vi "SetGXMLCfgRTD.vi"(8 "error in (no error)":errorcluster, 10 "RTDChanCfg":T1, 11 "RTD in":refnum<class "RTD.lvclass">) -> (0 "error out":errorcluster, 3 "RTD out":refnum<class "RTD.lvclass">)   [LabVIEW 2012, in "Measurement Channels.lvlib" / "RTD.lvclass"]
uses:
  RTD.lvclass
  RTDProps_TD.ctl
  RTD.lvclass/RTD.ctl
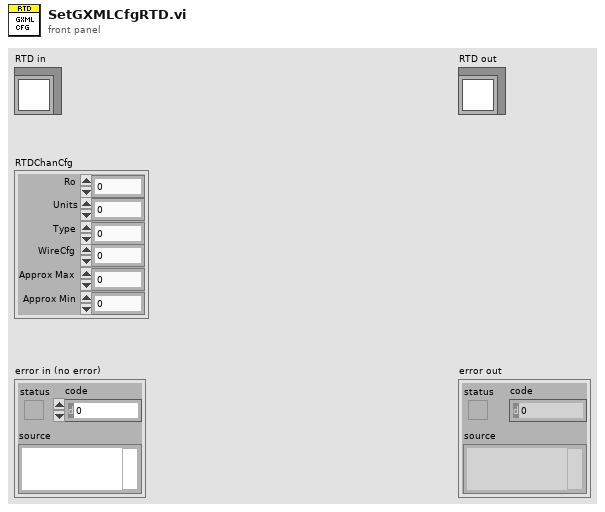
[diagram p1: front panel]
types:
  T1 = typedef "Measurement Channels.lvlib/RTD.lvclass/RTDProps_TD.ctl" = cluster{"Ro":u16, "Units":u16, "Type":u16, "WireCfg":u16, "Approx Max":dbl, "Approx Min":dbl}
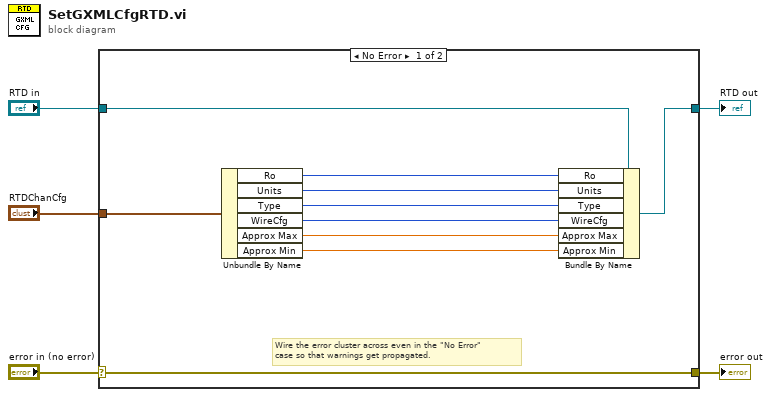
[diagram p0: block diagram]
diagram:
  n1 = case shown="No Error" "error in (no error)" {
    selector: "error in (no error)" -> [w15 w17]
    tunnel: [w15 w17] -> w4
    tunnel: [w7 w16] -> w2
    tunnel: "RTD in" -> [w8 w16]
    tunnel: "RTDChanCfg" -> [w6 _]
    frame No Error {
      # "Wire the error cluster across even in the \"No Error\"\ncase so that warnings get propagated."
      n2 = Unbundle By Name(w6) -> ("Ro"=w14:u16, "Units"=w13:u16, "Type"=w12:u16, "WireCfg"=w11:u16, "Approx Max"=w10:dbl, "Approx Min"=w9:dbl)
      n3 = Bundle By Name(cluster=w8, "Ro"=w14, "Units"=w13, "Type"=w12, "WireCfg"=w11, "Approx Max"=w10, "Approx Min"=w9) -> (w7:refnum<class "RTD.lvclass">)
    }
    frame Error {
    }
  }
  "error out" <- w4
  "RTD out" <- w2
